vi "Update.vi"(8 "error in (no error)":errorcluster, 11 "Deck in":refnum<class "Sample.lvclass">) -> (0 "error out":errorcluster, 2 "Audio Block":dbl[][](array[numeric]), 3 "Deck out":refnum<class "Sample.lvclass">)   [LabVIEW 2020, in "Sample.lvclass"]
uses:
  Sample.lvclass
  Sample.lvclass/Sample.ctl
  Packed Libraries/Globals.lvlibp/Constants.vi
  Packed Libraries/Messaging.lvlibp
  Packed Libraries/Globals.lvlibp
  Packed Libraries/Audio Processing.lvlibp
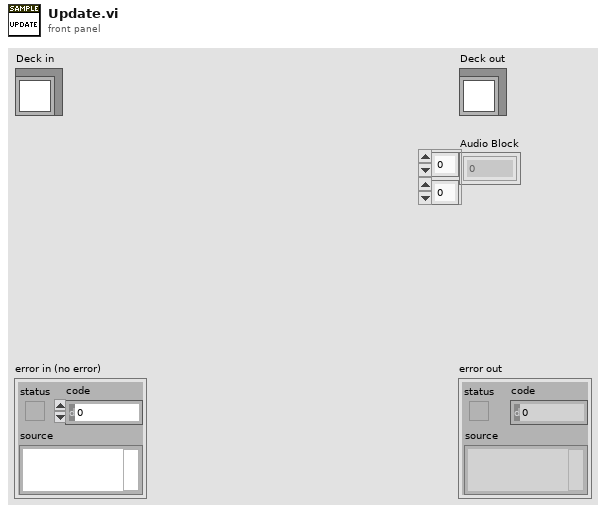
[diagram p1: front panel]
types:
  T1 = typedef "Sample.lvclass/State.ctl" = enum16{"No Track", "Loading", "Active", "Scratching", "Brake", "Backspin"}
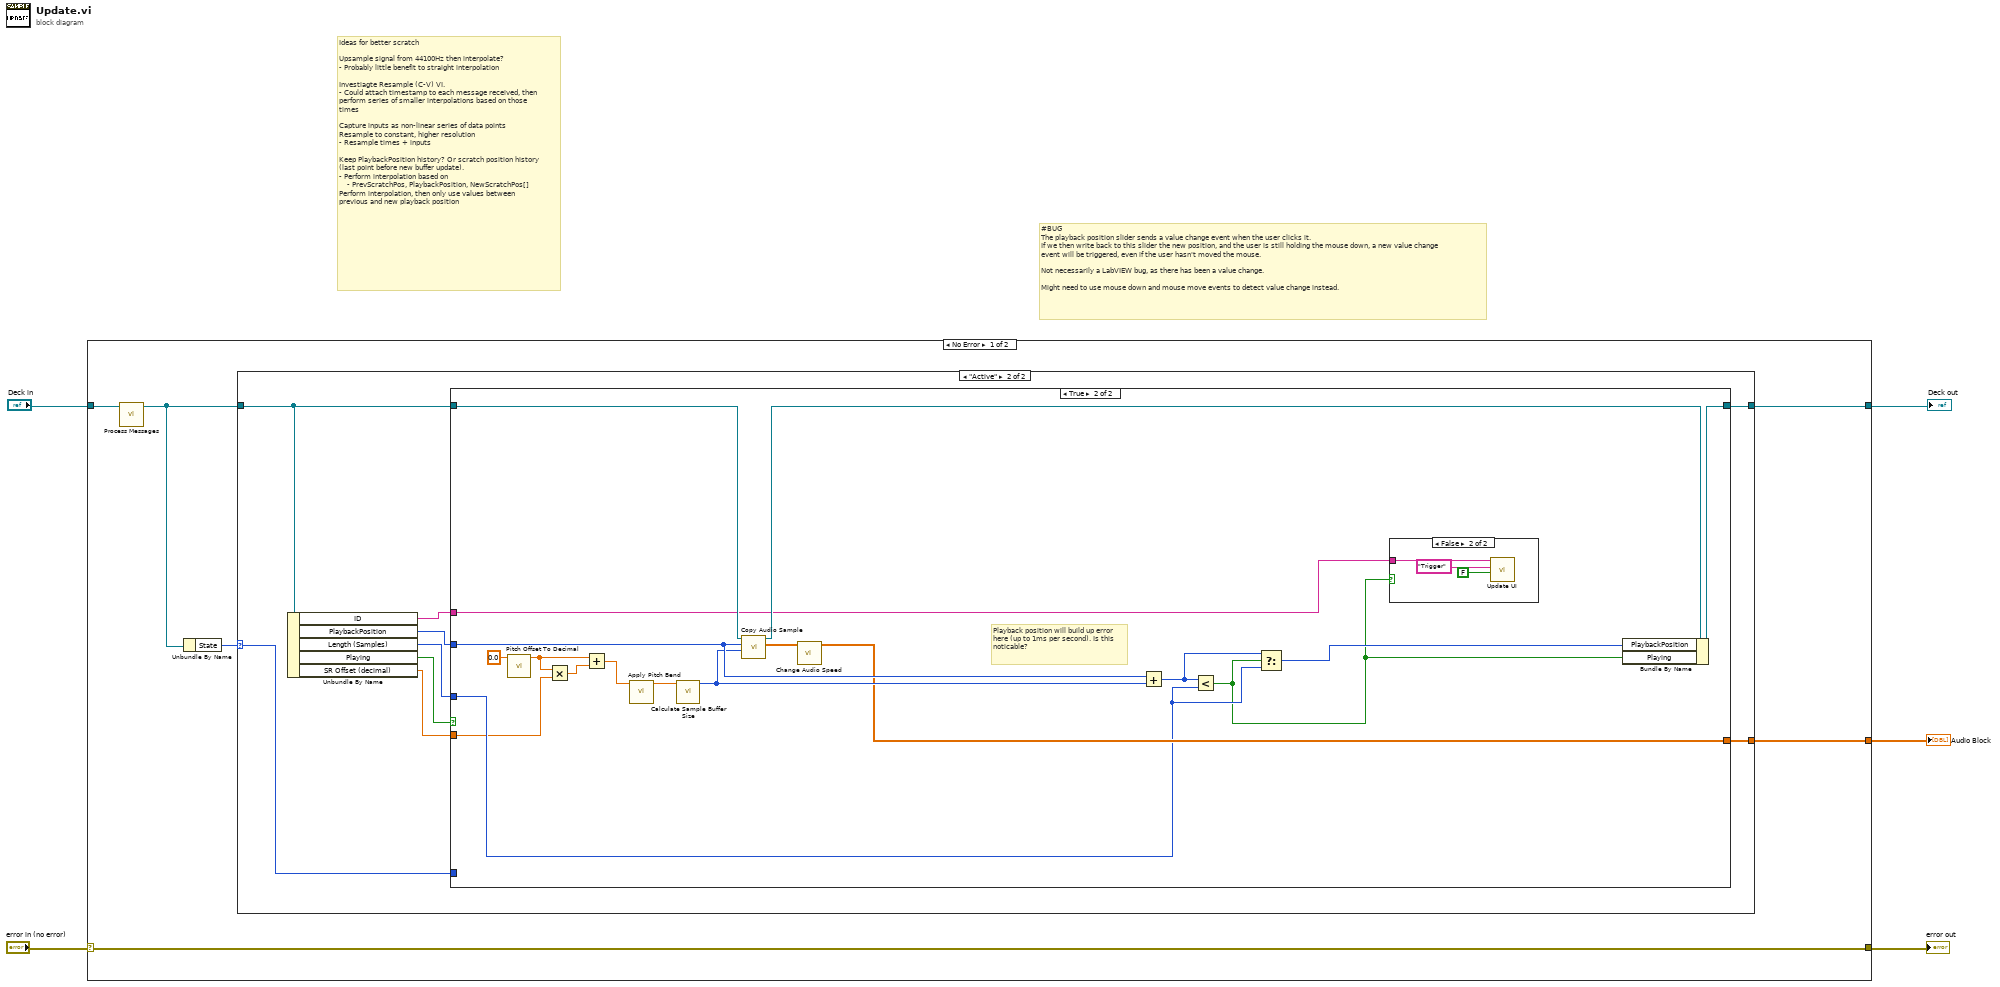
[diagram p0: block diagram]
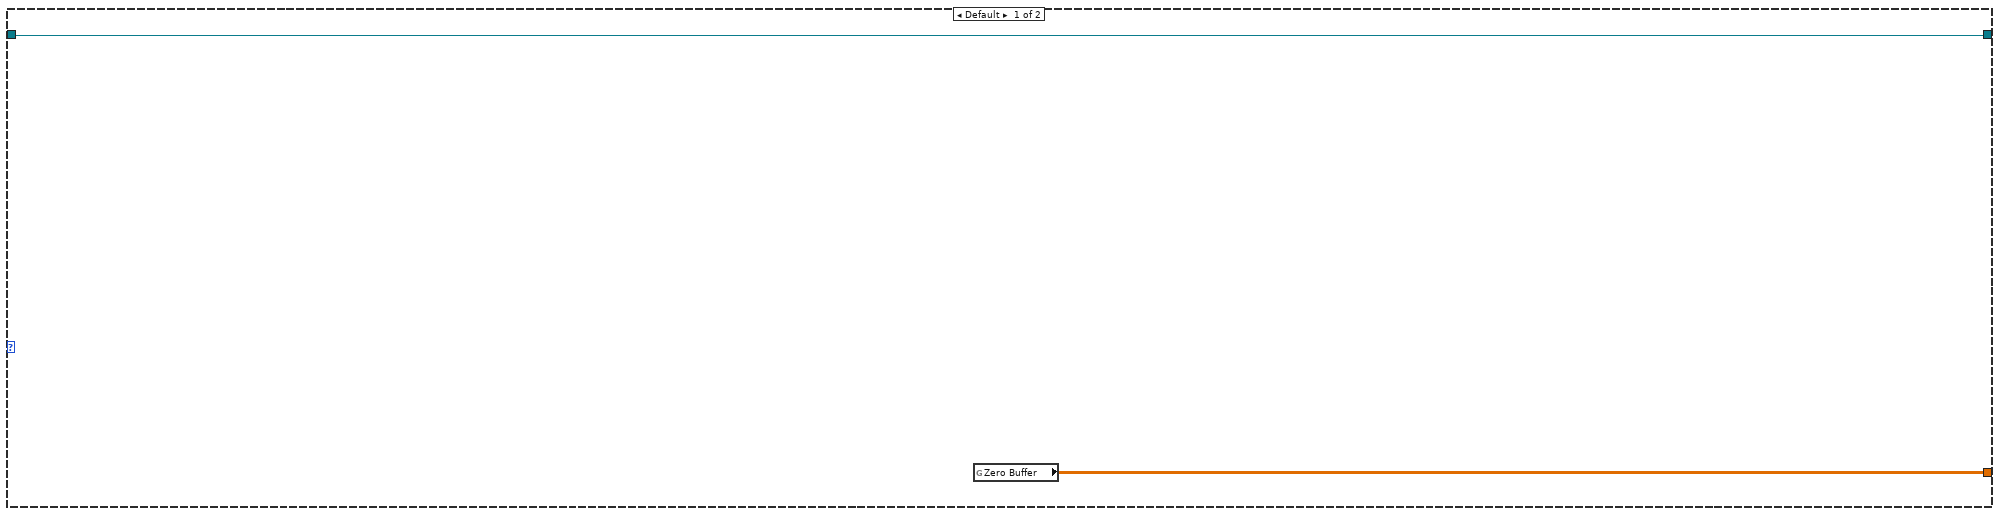
[diagram p2: hidden frame]
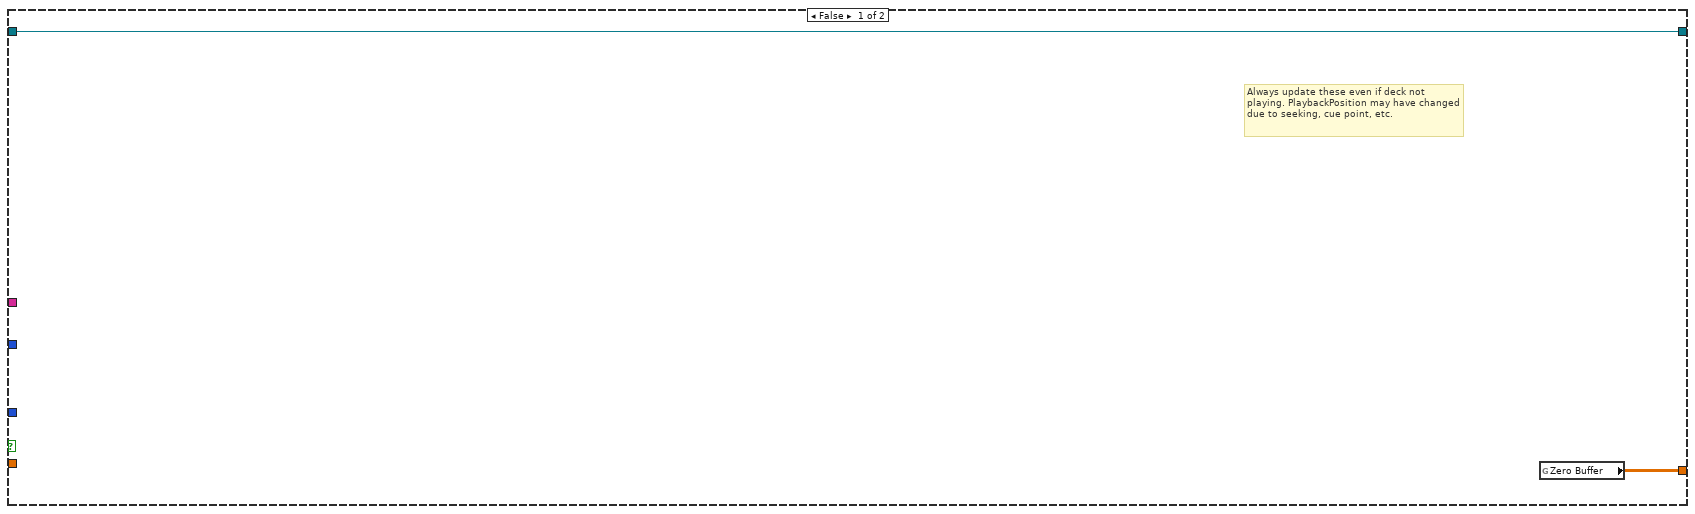
[diagram p3: hidden frame]
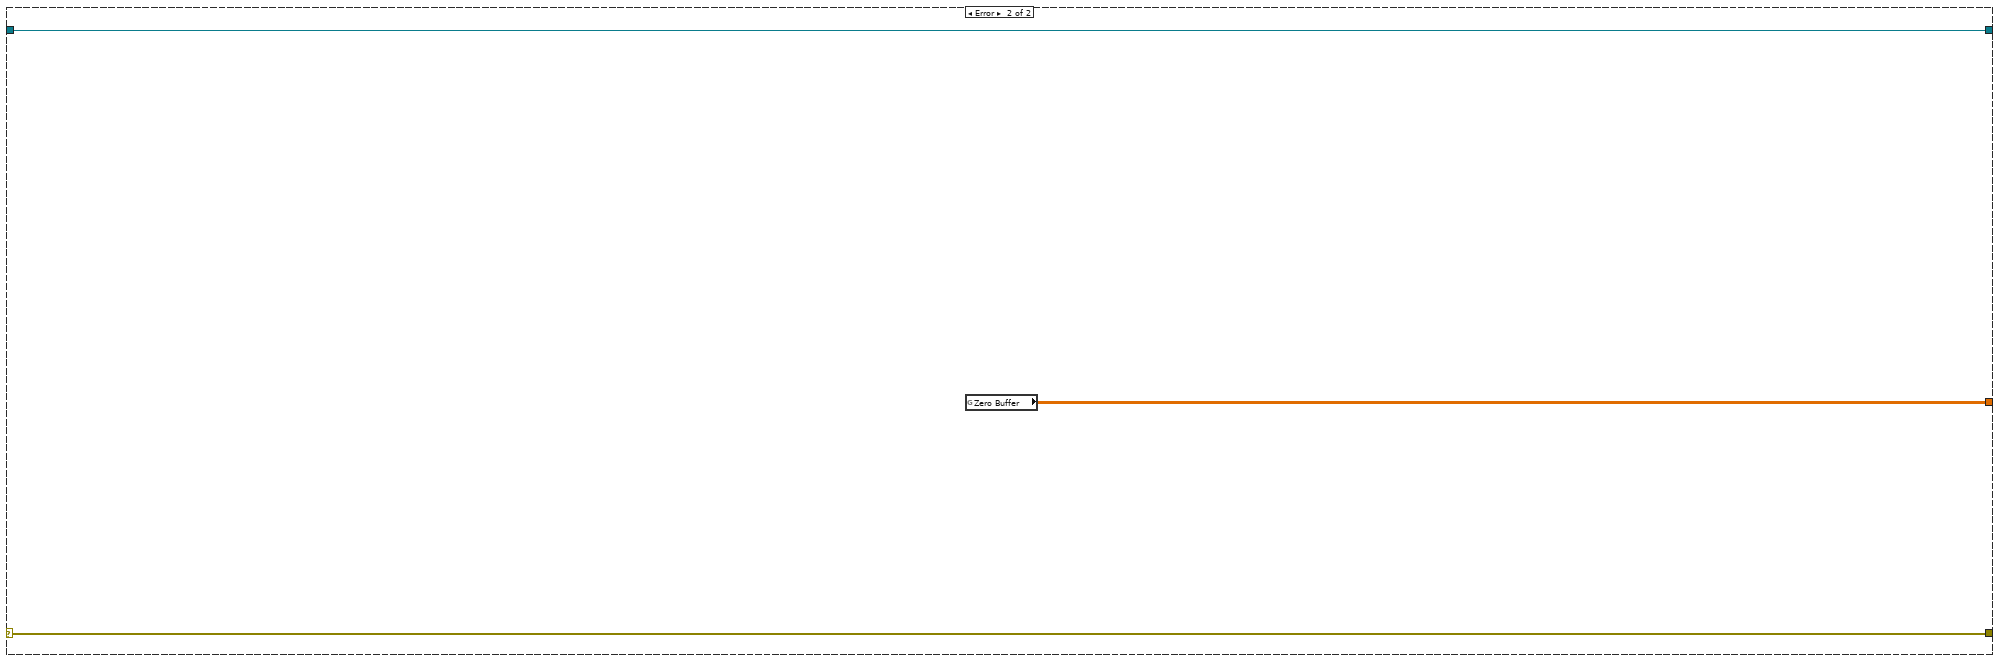
[diagram p5: hidden frame]
diagram:
  # "Ideas for better scratch\n\nUpsample signal from 44100Hz then interpolate?\n- Probably little benefit to straight interpolation\n\nInvestiagte Resample (C-V) VI.\n- Could attach timestamp to each message received, then perform series of smaller interpolations based on those times\n\nCapture inputs as non-linear series of data points\nResample to constant, higher resolution\n- Resample times + inputs\n\nKeep PlaybackPosition history? Or scratch position history (last point before new buffer update).\n- Perform interpolation based on\n    - PrevScratchPos, PlaybackPosition, NewScratchPos[]\nPerform interpolation, then only use values between previous and new playback position"
  # "#BUG\nThe playback position slider sends a value change event when the user clicks it.\nIf we then write back to this slider the new position, and the user is still holding the mouse down, a new value change event will be triggered, even if the user hasn't moved the mouse.\n\nNot necessarily a LabVIEW bug, as there has been a value change.\n\nMight need to use mouse down and mouse move events to detect value change instead."
  n1 = case shown="No Error" "error in (no error)" {
    selector: "error in (no error)" -> [w11 w48]
    tunnel: [w11 w48] -> w4
    tunnel: [w9 w47] -> w2
    tunnel: "Deck in" -> [w6 w47]
    tunnel: [w8 w46] -> w1
    frame No Error {
      n2 = call "Process Messages.vi"("Deck in"=w6) -> ("Deck out"=w7:refnum<class "Sample.lvclass">)  [unwired: 9 in, 1 out]
      n3 = Unbundle By Name(w7) -> ("State"=w10:T1)
      n4 = case shown="\"Active\"" w10 {
        selector: w10 -> [_ w18]
        tunnel: [w13 w22] -> w9
        tunnel: w7 -> [w13 w21]
        tunnel: [w12 w19] -> w8
        frame Default {
          n5 = global read "Constants.vi" "Zero Buffer"() -> (w12:dbl[][])
        }
        frame "Active" {
          n6 = Unbundle By Name(w21) -> ("ID"=w15:string, "PlaybackPosition"=w20:i32, "Length (Samples)"=w17:i32, "Playing"=w16:bool, "SR Offset (decimal)"=w14:dbl)
          n7 = case shown="True" w16 {
            tunnel: [w23 w42] -> w22
            tunnel: w21 -> [w23 w40]
            tunnel: w20 -> [_ w39]
            tunnel: [w24 w36] -> w19
            tunnel: w18 -> [_ _]
            tunnel: w15 -> [_ w31]
            tunnel: w17 -> [_ w35]
            tunnel: w14 -> [_ w28]
            frame False {
              # "Always update these even if deck not playing. PlaybackPosition may have changed due to seeking, cue point, etc."
              n8 = global read "Constants.vi" "Zero Buffer"() -> (w24:dbl[][])
            }
            frame True {
              # "Playback position will build up error here (up to 1ms per second). Is this noticable?"
              n9 = call "Pitch Offset To Decimal.vi"("Pitch Offset (%)"=0.0) -> ("Pitch (decimal)"=w27:dbl)  [unwired: 10 in]
              n10 = Multiply(x=w27, y=w28) -> (x*y=w26:dbl)
              n11 = Add(x=w27, y=w26) -> (x+y=w30:dbl)
              n12 = call "Apply Pitch Bend.vi"("Pitch (decimal) In"=w30) -> ("Pitch (decimal) Out"=w29:dbl)  [unwired: 10 in]
              n13 = call "Calculate Sample Buffer Size.vi"("Speed Multiplier"=w29) -> ("Sample Size"=w38:i32)  [unwired: 10 in]
              n14 = call "Copy Audio Sample.vi"("Length"=w38, "Offset"=w39, "Deck in"=w40) -> ("Audio Block"=w37:dbl[][], "Deck out"=w41:refnum<class "Sample.lvclass">)  [unwired: 6 in, 1 out]
              n15 = call "Change Audio Speed.vi"("Audio Block"=w37) -> ("Interpolated Audio"=w36:dbl[][])  [unwired: 10 in]
              n16 = Add(x=w39, y=w38) -> (x+y=w34:i32)
              n17 = Less?(x=w34, y=w35) -> (x < y?=w32:bool)
              n18 = Select(t=w34, s=w32, f=w35) -> (s? t:f=w33:i32)
              n19 = case shown="False" w32 {
                tunnel: w31 -> [_ w43]
                frame True {
                }
                frame False {
                  n20 = call "Update UI.vi"("Data"=FALSE, "Target"="Trigger" ("format string"), "ID"=w43) -> ()  [unwired: 8 in, 1 out]
                }
              }
              n21 = Bundle By Name(cluster=w41, "PlaybackPosition"=w33, "Playing"=w32) -> (w42:refnum<class "Sample.lvclass">)
            }
          }
        }
      }
    }
    frame Error {
      n22 = global read "Constants.vi" "Zero Buffer"() -> (w46:dbl[][])
    }
  }
  "error out" <- w4
  "Deck out" <- w2
  "Audio Block" <- w1
